vi "panel_update_status_string.vi"(8 "error in (no error)":errorcluster, 10 "String":string, 11 "hydraharp_panel in":refnum<class "hydraharp_panel.lvclass">) -> (0 "error out":errorcluster, 3 "hydraharp_panel out":refnum<class "hydraharp_panel.lvclass">)   [LabVIEW 2015, in "hydraharp_panel.lvclass"]
uses:
  hydraharp_panel.lvclass
  hydraharp_panel.lvclass/hydraharp_panel.ctl
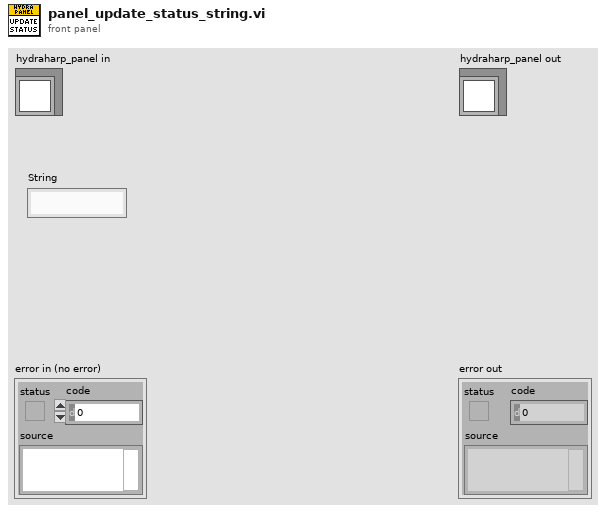
[diagram p1: front panel]
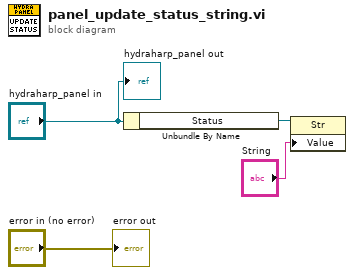
[diagram p0: block diagram]
diagram:
  n1 = Unbundle By Name("hydraharp_panel in") -> ("Status"=w4:refnum<vi>)
  n2 = property class="Str"(reference=w4, "Value"="String") -> ()  [unwired: 1 in, 2 out]
  "error out" <- "error in (no error)"
  "hydraharp_panel out" <- "hydraharp_panel in"
